vi "roller_read_sws.vi"(11 "output cluster":T5) -> (3 "sws":T1)   [LabVIEW 2011]
uses:
  <vilib>/Rock Robotics/WPI/DigitalInput/WPI_DigitalInputDevRef.ctl
  <vilib>/Rock Robotics/SystemInterfaces/DIO/FPGA_DIOChannel.ctl
  <vilib>/Rock Robotics/SystemInterfaces/Typedef/FPGA_TypedefDigitalModule.ctl
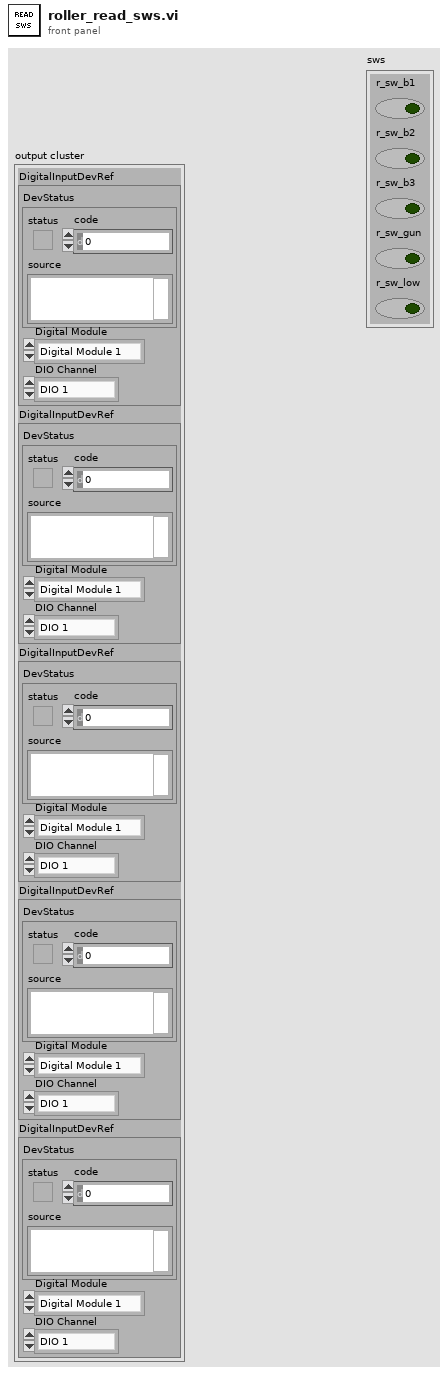
[diagram p1: front panel]
types:
  T1 = cluster{"r_sw_b1":bool, "r_sw_b2":bool, "r_sw_b3":bool, "r_sw_gun":bool, "r_sw_low":bool}
  T2 = typedef "WPI_DigitalInputDevRef.ctl" = cluster{"DevStatus":errorcluster, "DIO Channel":T3, "Digital Module":T4}
  T3 = typedef "FPGA_DIOChannel.ctl" = enum8{"DIO 1", "DIO 2", "DIO 3", "DIO 4", "DIO 5", "DIO 6", "DIO 7", "DIO 8", "DIO 9", "DIO 10", "DIO 11", "DIO 12", "DIO 13", "DIO 14", "Invalid"}
  T4 = typedef "FPGA_TypedefDigitalModule.ctl" = enum16{"Digital Module 1", "Digital Module 2"}
  T5 = cluster{"DigitalInputDevRef":T2, "DigitalInputDevRef":T2, "DigitalInputDevRef":T2, "DigitalInputDevRef":T2, "DigitalInputDevRef":T2}
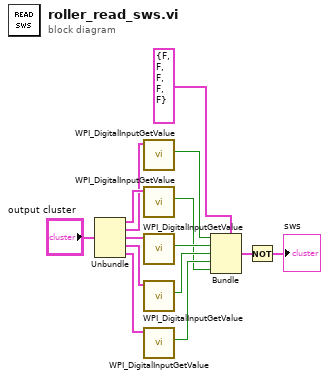
[diagram p0: block diagram]
diagram:
  n1 = Unbundle("output cluster") -> ("DigitalInputDevRef"=w12:T2, "DigitalInputDevRef"=w9:T2, "DigitalInputDevRef"=w8:T2, "DigitalInputDevRef"=w7:T2, "DigitalInputDevRef"=w6:T2)
  n2 = call <vilib>:"WPI_DigitalInputGetValue.vi"("DigitalInputDevRef"=w9) -> ("Value"=w5:bool)  [unwired: 8 in, 2 out]
  n3 = call <vilib>:"WPI_DigitalInputGetValue.vi"("DigitalInputDevRef"=w12) -> ("Value"=w1:bool)  [unwired: 8 in, 2 out]
  n4 = call <vilib>:"WPI_DigitalInputGetValue.vi"("DigitalInputDevRef"=w8) -> ("Value"=w4:bool)  [unwired: 8 in, 2 out]
  n5 = call <vilib>:"WPI_DigitalInputGetValue.vi"("DigitalInputDevRef"=w7) -> ("Value"=w3:bool)  [unwired: 8 in, 2 out]
  n6 = call <vilib>:"WPI_DigitalInputGetValue.vi"("DigitalInputDevRef"=w6) -> ("Value"=w2:bool)  [unwired: 8 in, 2 out]
  n7 = Bundle(cluster=T1 {"r_sw_b1"=FALSE, "r_sw_b2"=FALSE, "r_sw_b3"=FALSE, "r_sw_gun"=FALSE, "r_sw_low"=FALSE} ("sws"), "r_sw_b1"=w5, "r_sw_b2"=w4, "r_sw_b3"=w3, "r_sw_gun"=w2, "r_sw_low"=w1) -> (w11:T1)
  n8 = Not(x=w11) -> (.not. x?=→"sws":T1)
